vi "Actor Core.vi"(8 "error in":errorcluster, 11 "Example GUI Container in":refnum<class "Example GUI Container.lvclass">) -> (0 "error out":errorcluster, 3 "Actor out":refnum<class "Actor.lvclass">)   [LabVIEW 2017, in "Example GUI View Actor.lvlib" / "Example GUI Container.lvclass"]
doc: "(<B>Filename</B>: Actor Framework.lvlib:Actor.lvclass:Actor Core.vi)\n\nReceives messages to the actor, reacts to them, and initiates any error handling that may shut the actor down.\n\nDescendant classes may override this VI to append parallel tasks for the actor to complete while it handles messages. Overrides use the Call Parent Method node."
uses:
  Example GUI Container.lvclass
  C:/Projects/Shared Libraries/Event Actors/GUI Views/GUI Container Actor/GUI Container Actor.lvclass
  C:/Program Files (x86)/National Instruments/LabVIEW 2017/vi.lib/ActorFramework/Actor/Actor.lvclass
  <vilib>/ActorFramework/Actor/Actor.lvclass
  <vilib>/ActorFramework/Actor/Actor.lvclass/Actor.ctl
  <vilib>/ActorFramework/Message Enqueuer/Message Enqueuer.lvclass/Message Enqueuer.ctl
  <vilib>/ActorFramework/Message Enqueuer/Init from Existing Queue.vi
  <vilib>/ActorFramework/Message Enqueuer/Enqueue.vi
  <vilib>/ActorFramework/Stop Msg/Stop Msg.lvclass
  C:/Program Files (x86)/National Instruments/LabVIEW 2017/vi.lib/ActorFramework/Message/Message.lvclass
  <vilib>/Utility/LVClass/Get LV Class Name.vi
  <resource>/AFDebug/Generate Trace for Message.vi
  <vilib>/ActorFramework/Message Priority Queue/Priority Enqueue.vi
  <vilib>/ActorFramework/Message Enqueuer/Message Enqueuer.lvclass
  GUI Views/GUI Container Actor/GUI Container Actor.lvclass
  GUI Views/GUI Container Actor Messages/Read Views Msg/Read Views Msg.lvclass
  GUI Views/GUI Container Actor Messages/Insert View into Subpanel Msg/Insert View into Subpanel Msg.lvclass
  GUI Views/GUI Container Actor Messages/Set View FP State Msg/Set View FP State Msg.lvclass
  GUI Views/GUI Container Actor Messages/Open View FP Msg/Open View FP Msg.lvclass
  GUI Views/GUI Container Actor Messages/Close View FP Msg/Close View FP Msg.lvclass
  GUI Views/GUI Container Actor Messages/Remove View from Subpanel Msg/Remove View from Subpanel Msg.lvclass
panel:
  in  "Remove from Subpanel":bool
  in  "Subpanel":string(combo)
  in  "Close Front Panel":bool
  in  "Activate on Open (F)":bool
  in  "Open Front Panel":bool
  in  "Front Panel State":T1(ring)=enum."Standard"
  in  "Set FP State":bool
  in  "Insert in Subpanel":bool
  in  "Exit":bool
  in  "Views":i32(listbox)
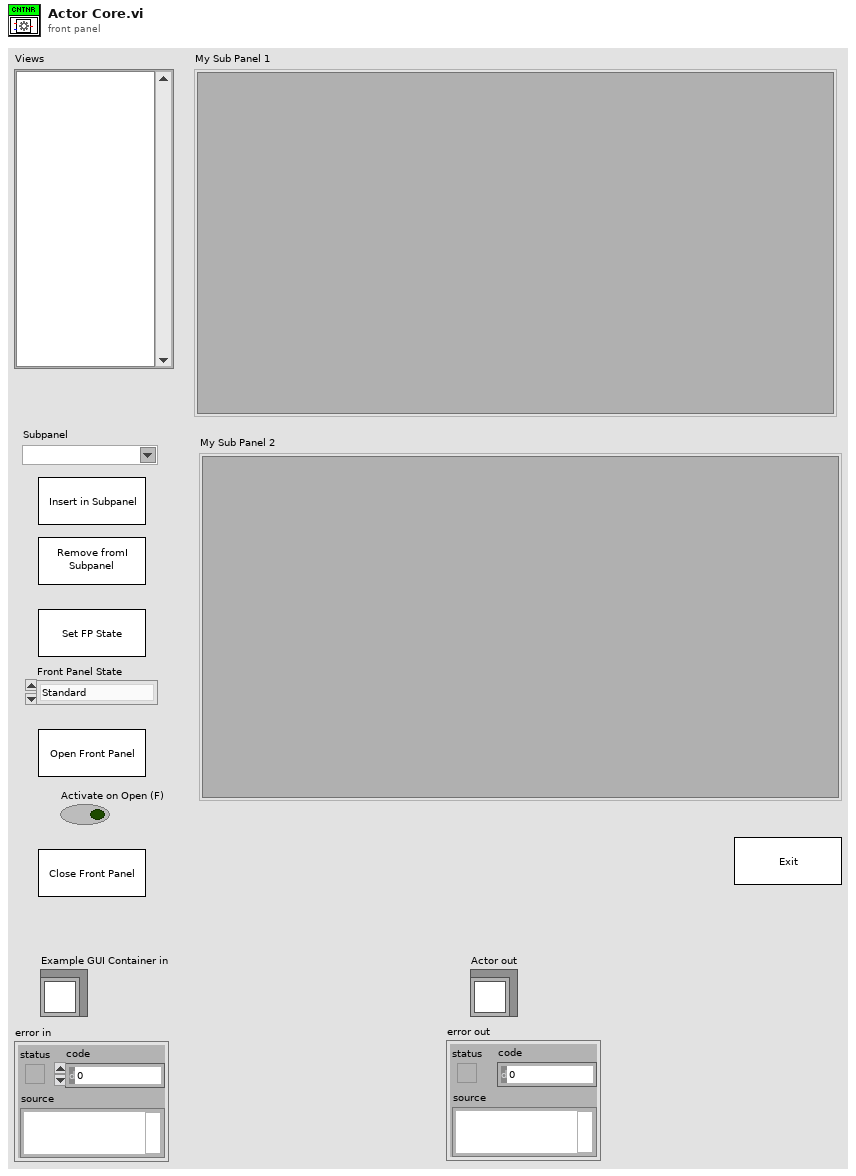
[diagram p1: front panel]
types:
  T1 = enum32{"Invalid", "Standard", "Closed", "Hidden", "Minimized", "Maximized"}
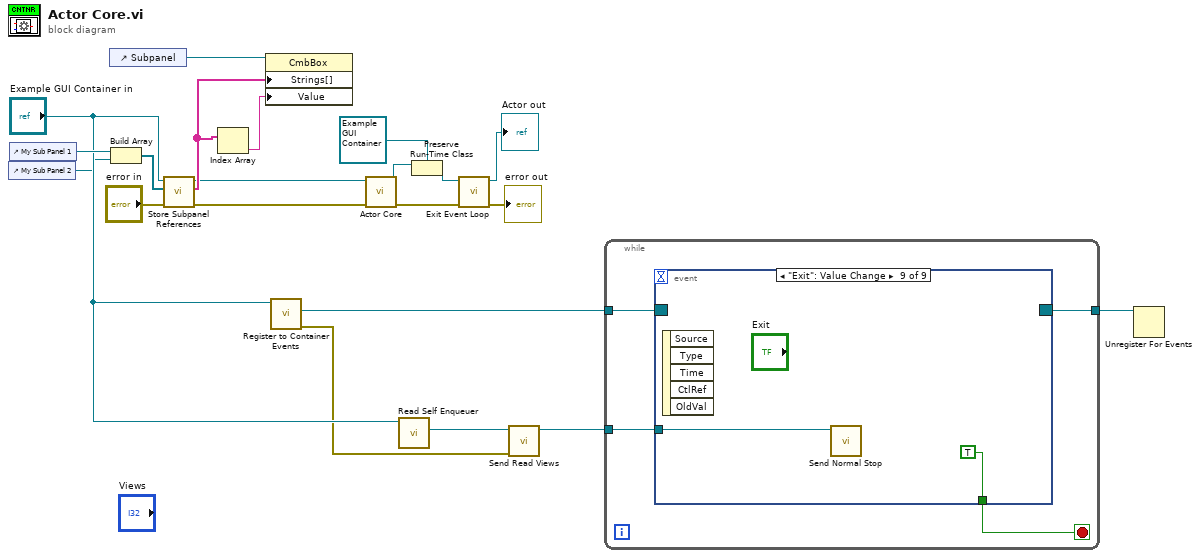
[diagram p0: block diagram]
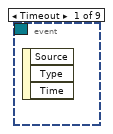
[diagram p2: hidden frame]
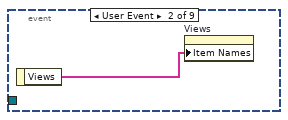
[diagram p3: hidden frame]
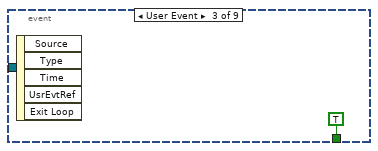
[diagram p4: hidden frame]
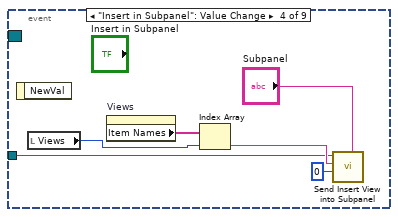
[diagram p5: hidden frame]
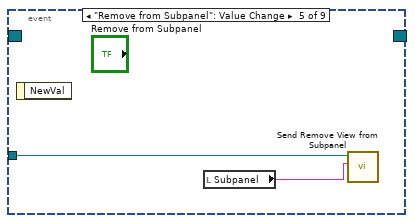
[diagram p6: hidden frame]
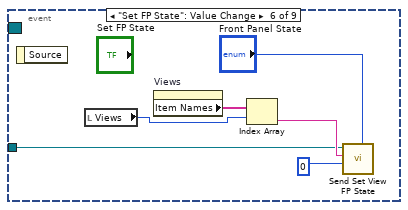
[diagram p7: hidden frame]
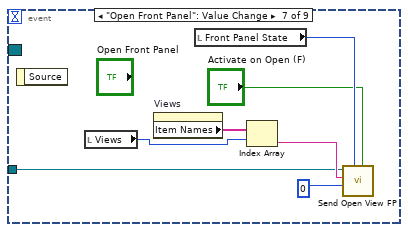
[diagram p8: hidden frame]
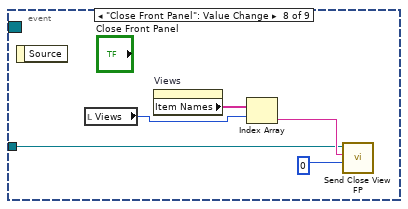
[diagram p9: hidden frame]
diagram:
  n1 = control-ref of="My Sub Panel 2"() -> (w11:refnum<vi>)
  n2 = control-ref of="My Sub Panel 1"() -> (w21:refnum<vi>)
  n3 = control-ref of="Subpanel"() -> (w10:refnum<vi>)
  n4 = Build Array(w21, w11) -> (w20:refnum<vi>[])
  n5 = call "Store Subpanel References.vi"("error in (no error)"="error in", "Subpanel References"=w20, "GUI Container Actor in"="Example GUI Container in") -> ("error out"=w18:errorcluster, "Sub Panel Names"=w9:string[], "GUI Container Actor out"=w6:refnum<class "Example GUI Container.lvclass">)  [unwired: 6 in]
  n6 = Index Array(array=w9) -> (element=w8:string)  [unwired: 1 in]
  n7 = property class="CmbBox"(reference=w10, "Strings[]"=w9, "Value"=w8) -> ()  [unwired: 1 in, 2 out]
  n8 = call-dynamic "Register to Container Events.vi"("GUI Container Actor in"="Example GUI Container in") -> ("error out"=w14:errorcluster, "Event Registration Refnum"=w17:refnum<event-registration>)  [unwired: 8 in, 1 out]
  n9 = call-parent "Actor Core.vi"("error in"=w18, "GUI View Actor in"=w6) -> ("error out"=w4:errorcluster, "Actor out"=w7:refnum<class "Actor.lvclass">)  [unwired: 8 in]
  n10 = call <vilib>:"Read Self Enqueuer.vi"("Actor"="Example GUI Container in") -> ("Self Enqueuer"=w15:refnum<class "Message Enqueuer.lvclass">)  [unwired: 10 in]
  n11 = Preserve Run-Time Class(object in=w7, 2:refnum<class "Example GUI Container.lvclass"> refnum ("Example GUI Container in")) -> (object out=w5:refnum<class "Example GUI Container.lvclass">)  [unwired: 1 in, 1 out]
  n12 = call "Exit Event Loop.vi"("error in (no error)"=w4, "GUI Container Actor in"=w5) -> ("error out"=→"error out":errorcluster, "GUI Container Actor out"=→"Actor out":refnum<class "Example GUI Container.lvclass">)  [unwired: 8 in]
  n13 = call "Send Read Views.vi"("error in (no error)"=w14, "Message Enqueuer in"=w15) -> ("Message Enqueuer out"=w13:refnum<class "Message Enqueuer.lvclass">)  [unwired: 8 in, 1 out]
  n14 = while {
    tunnel: w17 -> [w25]
    tunnel: w13 -> [w24]
    tunnel: [w22] -> w12
    stop <- w23 stop-if-true
    n15 = event shown="[8] \"Exit\": Value Change" {
      selector: w25 -> [_ _ _ _ _ _ _ _ _]
      dyn-events: [_ _ _ _ _ _ _ _ _] -> w22
      timeout: _ -> [_ _ _ _ _ _ _ _ _]
      tunnel: w24 -> [_ _ _ w30 w34 w38 w45 w50 w55]
      tunnel: [_ _ TRUE _ _ _ _ _ TRUE] -> w23
      event Timeout {
        n16 = event-data() -> ()  [unwired: 1 in, 3 out]
      }
      event User Event {
        n17 = event-data() -> ("Views"=w26:string[])  [unwired: 1 in]
        n18 = property on="Views" class="LstBox (strict)"("Item Names"=w26) -> ()  [unwired: 2 in, 2 out]
      }
      event User Event {
        n19 = event-data() -> ()  [unwired: 1 in, 5 out]
      }
      event "Insert in Subpanel": Value Change {
        n20 = event-data() -> ()  [unwired: 1 in, 1 out]
        n21 = local read "Views"() -> (w29:i32)
        n22 = property on="Views" class="LstBox (strict)"() -> ("Item Names"=w33:string[])  [unwired: 2 in, 2 out]
        n23 = Index Array(array=w33, index=w29) -> (element=w32:string)
        n24 = call "Send Insert View into Subpanel.vi"("Subpanel"="Subpanel", "View Hierarchy Level"=0, "View"=w32, "Message Enqueuer in"=w30) -> ()  [unwired: 6 in, 2 out]
      }
      event "Remove from Subpanel": Value Change {
        n25 = event-data() -> ()  [unwired: 1 in, 1 out]
        n26 = local read "Subpanel"() -> (w35:string)
        n27 = call "Send Remove View from Subpanel.vi"("Subpanel"=w35, "Message Enqueuer in"=w34) -> ()  [unwired: 8 in, 2 out]
      }
      event "Set FP State": Value Change {
        n28 = event-data() -> ()  [unwired: 1 in, 1 out]
        n29 = local read "Views"() -> (w36:i32)
        n30 = property on="Views" class="LstBox (strict)"() -> ("Item Names"=w41:string[])  [unwired: 2 in, 2 out]
        n31 = Index Array(array=w41, index=w36) -> (element=w40:string)
        n32 = call "Send Set View FP State.vi"("Front Panel Window:State"="Front Panel State", "View Hierarchy Level"=0, "View"=w40, "Message Enqueuer in"=w38) -> ()  [unwired: 6 in, 2 out]
      }
      event "Open Front Panel": Value Change {
        n33 = event-data() -> ()  [unwired: 1 in, 1 out]
        n34 = local read "Views"() -> (w44:i32)
        n35 = property on="Views" class="LstBox (strict)"() -> ("Item Names"=w48:string[])  [unwired: 2 in, 2 out]
        n36 = local read "Front Panel State"() -> (w43:T1)
        n37 = Index Array(array=w48, index=w44) -> (element=w47:string)
        n38 = call "Send Open View FP.vi"("Activate on Open (F)"="Activate on Open (F)", "State On Open (Standard)"=w43, "View Hierarchy Level"=0, "View"=w47, "Message Enqueuer in"=w45) -> ()  [unwired: 5 in, 2 out]
      }
      event "Close Front Panel": Value Change {
        n39 = event-data() -> ()  [unwired: 1 in, 1 out]
        n40 = local read "Views"() -> (w49:i32)
        n41 = property on="Views" class="LstBox (strict)"() -> ("Item Names"=w53:string[])  [unwired: 2 in, 2 out]
        n42 = Index Array(array=w53, index=w49) -> (element=w52:string)
        n43 = call "Send Close View FP.vi"("View Hierarchy Level"=0, "View"=w52, "Message Enqueuer in"=w50) -> ()  [unwired: 7 in, 2 out]
      }
      event "Exit": Value Change {
        n44 = event-data() -> ()  [unwired: 1 in, 5 out]
        n45 = call <vilib>:"Send Normal Stop.vi"("Message Enqueuer"=w55) -> ()  [unwired: 10 in, 1 out]
      }
    }
  }
  n46 = Unregister For Events(event registration refnum=w12) -> ()  [unwired: 1 in, 1 out]
